vi "open.vi"(8 "error in (no error)":errorcluster caption="错误输入（无错误）", 11 "GPS 输入":refnum<class "GPS.lvclass">) -> (0 "error out":errorcluster caption="错误输出", 3 "GPS 输出":refnum<class "GPS.lvclass">)   [LabVIEW 2016, in "GPS.lvlib" / "GPS.lvclass"]
uses:
  GPS.lvclass
  GPS.lvclass/GPS.ctl
  <vilib>/Instr/_visa.llb/VISA Configure Serial Port (Instr).vi
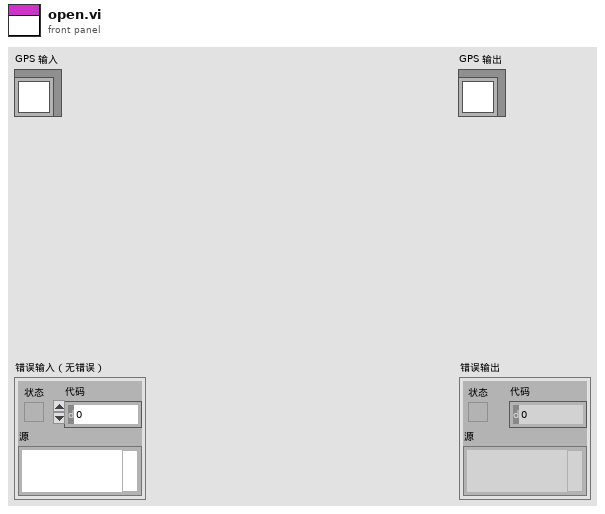
[diagram p1: front panel]
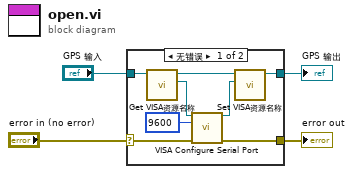
[diagram p0: block diagram]
diagram:
  n1 = case shown="无错误" "error in (no error)" {
    selector: "error in (no error)" -> [w9 w14]
    tunnel: [w5 w14] -> w3
    tunnel: [w6 w13] -> w1
    tunnel: "GPS 输入" -> [w12 w13]
    frame No Error {
      n2 = call "Get VISA资源名称.vi"("GPS in"=w12) -> ("VISA资源名称"=w11:refnum<visa-resource-name>, "GPS out"=w8:refnum<class "GPS.lvclass">)  [unwired: 9 in]
      n3 = call-poly "VISA Configure Serial Port"("VISA resource name"=w11, "baud rate (9600)"=u32 9600, "error in (no error)"=w9) -> ("VISA resource name out"=w7:refnum<visa-resource-name>, "error out"=w5:errorcluster)  [unwired: 11 in]
      n4 = call "Set VISA资源名称.vi"("VISA资源名称"=w7, "GPS in"=w8) -> ("GPS out"=w6:refnum<class "GPS.lvclass">)  [unwired: 9 in]
    }
    frame Error {
    }
  }
  "error out" <- w3
  "GPS 输出" <- w1
